vi "WebDevHost.vi"(11 "DataExport":bool) -> (1 "error out":errorcluster)   [LabVIEW 2020]
uses:
  <vilib>/WebDAVClient/Advanced/Get File.vi
  <vilib>/WebDAVClient/NI_WebDAV.lvlib
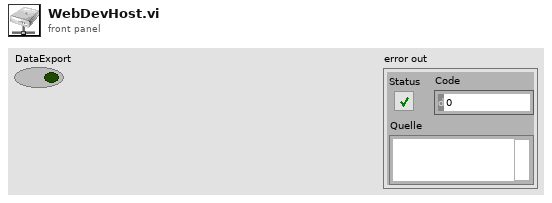
[diagram p1: front panel]
types:
  T1 = typedef "NI_WebDAV.lvlib/SessionHandle.ctl" = refnum<k1>
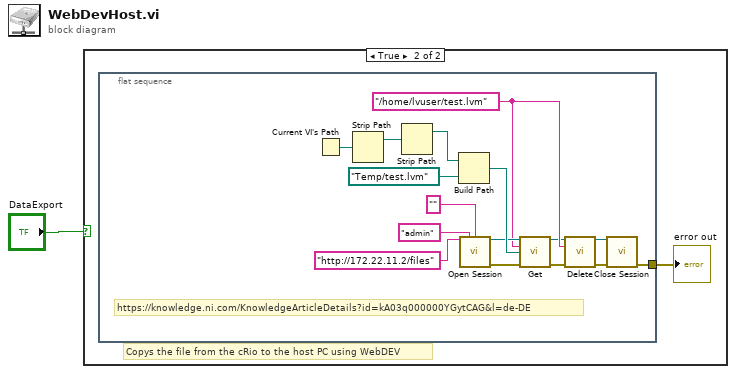
[diagram p0: block diagram]
diagram:
  n1 = case shown="True" "DataExport" {
    frame False {
    }
    frame True {
      # "Copys the file from the cRio to the host PC using WebDEV"
      n2 = flat-sequence {
        tunnel: [w15] -> w2
        frame #0 {
          w7 = "/home/lvuser/test.lvm" ("relative destination uri")
          # "https://knowledge.ni.com/KnowledgeArticleDetails?id=kA03q000000YGytCAG&l=de-DE"
          n3 = Current VI's Path() -> (path=w13:path)
          n4 = Strip Path(path=w13) -> (stripped path=w12:path)  [unwired: 1 out]
          n5 = Strip Path(path=w12) -> (stripped path=w11:path)  [unwired: 1 out]
          n6 = Build Path(base path=w11, name or relative path=path "Temp/test.lvm") -> (appended path=w9:path)
          n7 = call <vilib>:"Open Session.vi"("host uri prefix"="http://172.22.11.2/files", "username"="admin", "password"="") -> ("session handle out"=w8:T1, "error out"=w16:errorcluster)  [unwired: 11 in]
          n8 = call-poly <vilib>:"Get.vi"("session handle"=w8, "relative uri"=w7, "local file path"=w9, "error in (no error)"=w16) -> ("session handle out"=w6:T1, "error out"=w4:errorcluster)  [unwired: 9 in, 1 out]
          n9 = call <vilib>:"Delete.vi"("session handle"=w6, "relative uri"=w7, "error in (no error)"=w4) -> ("session handle out"=w5:T1, "error out"=w3:errorcluster)  [unwired: 11 in]
          n10 = call <vilib>:"Close Session.vi"("session handle"=w5, "error in (no error)"=w3) -> ("error out"=w15:errorcluster)  [unwired: 13 in]
        }
      }
      "error out" <- w2
    }
  }
